vi "Single_ITX_to_Wave_Info.vi"(8 "error in (no error)":errorcluster, 11 "Path":path) -> (0 "error out":errorcluster, 3 "Single ITX cluster":T1)   [LabVIEW 2016]
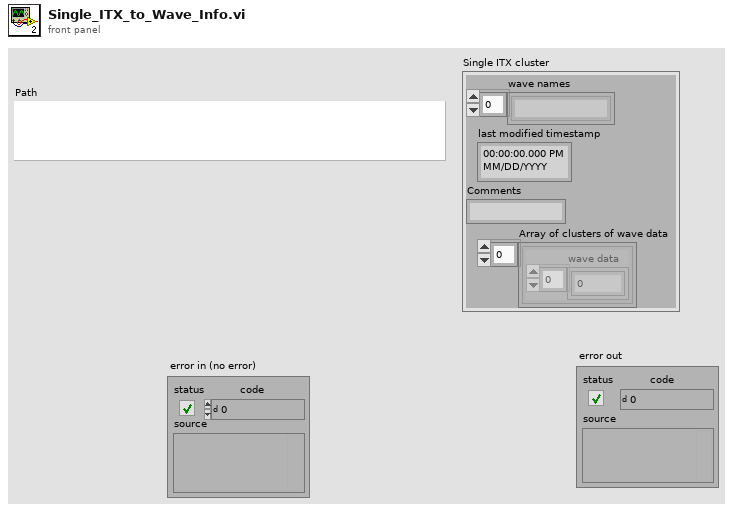
[diagram p1: front panel]
types:
  T1 = cluster{"wave names":string[], "last modified timestamp":timestamp, "Comments":string, "Array of clusters of wave data":cluster{"wave data":dbl[]}[]}
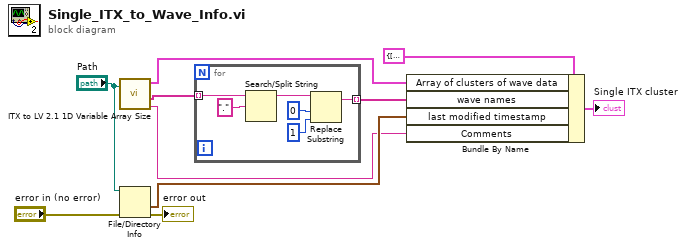
[diagram p0: block diagram]
diagram:
  n1 = call "ITX to LV 2.1 1D Variable Array Size.vi"("file (use dialog)"="Path") -> ("Array of clusters of wave data"=w4:cluster{"wave data":dbl[]}[], "wave names"=w3:string[], "Notes"=w2:string)  [unwired: 2 in]
  n2 = File/Directory Info(path="Path", error in="error in (no error)") -> (last mod=w10:timestamp, error out=→"error out":errorcluster)  [unwired: 5 out]
  n3 = for {
    tunnel: w3 -> [w16] mode=indexing
    tunnel: [w11] -> w8 mode=indexing
    n4 = Search/Split String(string=w16, search string/char (-)=".") -> (substring before match=w12:string)  [unwired: 1 in, 2 out]
    n5 = Replace Substring(2:1 ("length (len. of substring)"), 3:0 ("offset (0)"), 5:w12) -> (1:w11:string)  [unwired: 1 in, 1 out]
  }
  n6 = Bundle By Name(cluster=T1 {"wave names"=[], "last modified timestamp"=timestamp(0 s since 1904-01-01), "Comments"="IGOR\nX// Date: 7/13/2018 2:27 PM\nX// SA03036H\nX// sweep Vsg:-150mV to 600mV, 1mV steps\nX// B: 7T to -7T\nX// Vbg = -3.9V\nX// T: 50mK\nX// \nX// lockin\nX// \nX// I+/-: 2/3 3mV ac+ 250uV dc bias, 0.4 Hz\nX// V1+/-: 8/4\nX// V2+/- 6/28\nX// V3+/V3-: 27/8\nX// Vsg: 1\nX// Vbg :26\nX// \nX// tc 300ms order 2\nX// B= -0.000001\n\n\n\n\n\n\n\n\n\n\n\n\n\n\n\n\n\n\n\n\n\n\n\n\n\n\n\n\n\n\n\n\n\n\n\n\n\n\n\n\nX \nX Display/R 'time.SA03008H.000203'\nX AppendToGraph 'temp.SA03008H.000203'\nX AppendToGraph 'B.SA03008H.000203'\nX AppendToGraph 'Vsource.SA03008H.000203'\nX AppendToGraph 'Lockin0.SA03008H.000203'\nX AppendToGraph 'Lockin1.SA03008H.000203'\nX AppendToGraph 'Lockin2.SA03008H.000203'\nX AppendToGraph 'Lockin3.SA03008H.000203'\nX AppendToGraph 'Lockin4.SA03008H.000203'\nX AppendToGraph 'Lockin5.SA03008H.000203'\nX AppendToGraph 'B_rate.SA03008H.000203'\nX AppendToGraph 'DC0.SA03008H.000203'\nX AppendToGraph 'DC1.SA03008H.000203'\nX AppendToGraph 'DC2.SA03008H.000203'\nX AppendToGraph 'DC3.SA03008H.000203'\nX AppendToGraph 'DC4.SA03008H.000203'\nX AppendToGraph 'DC5.SA03008H.000203'\nX AppendToGraph 'DC6.SA03008H.000203'\nX AppendToGraph 'DC7.SA03008H.000203'\nX Label bottom \"x label\"\nX Label left \"y label\"\nX ModifyGraph rgb('time.SA03008H.000203')=(65280,0,0)\nX ModifyGraph rgb('temp.SA03008H.000203')=(65280,18432,0)\nX ModifyGraph rgb('B.SA03008H.000203')=(65280,36864,0)\nX ModifyGraph rgb('Vsource.SA03008H.000203')=(65280,55296,0)\nX ModifyGraph rgb('Lockin0.SA03008H.000203')=(57344,65280,0)\nX ModifyGraph rgb('Lockin1.SA03008H.000203')=(37376,65280,0)\nX ModifyGraph rgb('Lockin2.SA03008H.000203')=(18944,65280,0)\nX ModifyGraph rgb('Lockin3.SA03008H.000203')=(512,65280,0)\nX ModifyGraph rgb('Lockin4.SA03008H.000203')=(0,65280,17920)\nX ModifyGraph rgb('Lockin5.SA03008H.000203')=(0,65280,36352)\nX ModifyGraph rgb('B_rate.SA03008H.000203')=(0,65280,54784)\nX ModifyGraph rgb('DC0.SA03008H.000203')=(0,57856,65280)\nX ModifyGraph rgb('DC1.SA03008H.000203')=(0,39424,65280)\nX ModifyGraph rgb('DC2.SA03008H.000203')=(0,20992,65280)\nX ModifyGraph rgb('DC3.SA03008H.000203')=(0,2560,65280)\nX ModifyGraph rgb('DC4.SA03008H.000203')=(17408,0,65280)\nX ModifyGraph rgb('DC5.SA03008H.000203')=(35840,0,65280)\nX ModifyGraph rgb('DC6.SA03008H.000203')=(54272,0,65280)\nX ModifyGraph rgb('DC7.SA03008H.000203')=(65280,0,58368)\nX Legend/C/N=text0/J \"\\\\s('time.SA03008H.000203') time\\r\\\\s('temp.SA03008H.000203') temp\\r\\\\s('B.SA03008H.000203') B\\r\\\\s('Vsource.SA03008H.000203') Vsource\\r\\\\s('Lockin0.SA03008H.000203') Lockin0\\r\\\\s('Lockin1.SA03008H.000203') Lockin1\\r\\\\s('Lockin2.SA03008H.000203') Lockin2\\r\\\\s('Lockin3.SA03008H.000203') Lockin3\\r\\\\s('Lockin4.SA03008H.000203') Lockin4\\r\\\\s('Lockin5.SA03008H.000203') Lockin5\\r\\\\s('B_rate.SA03008H.000203') B_rate\\r\\\\s('DC0.SA03008H.000203') DC0\\r\\\\s('DC1.SA03008H.000203') DC1\\r\\\\s('DC2.SA03008H.000203') DC2\\r\\\\s('DC3.SA03008H.000203') DC3\\r\\\\s('DC4.SA03008H.000203') DC4\\r\\\\s('DC5.SA03008H.000203') DC5\\r\\\\s('DC6.SA03008H.000203') DC6\\r\\\\s('DC7.SA03008H.000203') DC7\"\nX ModifyGraph mirror(bottom)=1\nX ModifyGraph width=216\nX ModifyGraph height={Aspect,0.6}\nX ModifyGraph Log(bottom)=0\nX ModifyGraph Log(left)=0\nX \n", "Array of clusters of wave data"=[]}, "Array of clusters of wave data"=w4, "wave names"=w8, "last modified timestamp"=w10, "Comments"=w2) -> (→"Single ITX cluster":T1)
